vi "Read Dashboard Variables.vi"() -> ()   [LabVIEW 2018]
uses:
  <vilib>/Rock Robotics/Network Tables/NT Read Number.vi
  Framework/Robot Global Data.vi
panel:
  out "Hatch Extend Duration":dbl
  out "Hatch Extend Setpoint":dbl
  out "SlowModeSettings":i32=2
  out "MaxSpeedSlow":dbl=0.4
  out "SlowRate":dbl=1.0
  out "MaxTurnSlow":dbl=0.55
  out "MaxTurnRateSlow":dbl=20.0
  out "Cargo Stop Current":dbl
  out "Cargo Hold Duration":dbl
  out "Cheezy Drive Mode":u32=2
  out "Cargo Setpoint":dbl
  out "Elevator Duration":dbl
  out "Elevator Setpoint":dbl
  out "Pivot Right Setpoint":dbl
  out "Pivot Left Setpoint":dbl
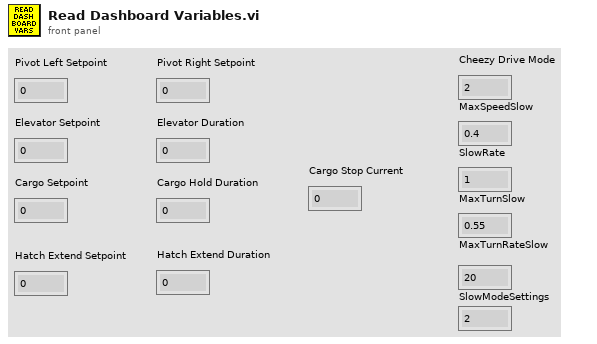
[diagram p1: front panel]
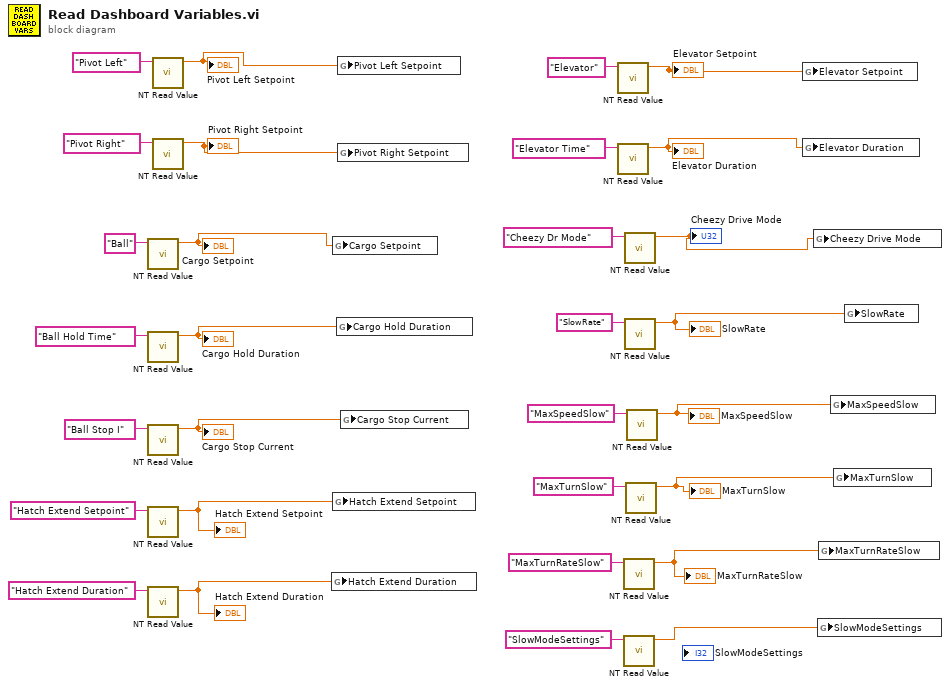
[diagram p0: block diagram]
diagram:
  n1 = call-poly <vilib>:"NT Read Value.vi"("Name"="Ball") -> ("Numeric"=w20:dbl)  [unwired: 9 in, 1 out]
  "Cargo Setpoint" <- w20
  n2 = call-poly <vilib>:"NT Read Value.vi"("Name"="Ball Hold Time") -> ("Numeric"=w18:dbl)  [unwired: 9 in, 1 out]
  "Cargo Hold Duration" <- w18
  n3 = call-poly <vilib>:"NT Read Value.vi"("Name"="Ball Stop I") -> ("Numeric"=w15:dbl)  [unwired: 9 in, 1 out]
  "Cargo Stop Current" <- w15
  n4 = call-poly <vilib>:"NT Read Value.vi"("Name"="Hatch Extend Setpoint") -> ("Numeric"=w2:dbl)  [unwired: 9 in, 1 out]
  "Hatch Extend Setpoint" <- w2
  n5 = call-poly <vilib>:"NT Read Value.vi"("Name"="Hatch Extend Duration") -> ("Numeric"=w1:dbl)  [unwired: 9 in, 1 out]
  "Hatch Extend Duration" <- w1
  n6 = call-poly <vilib>:"NT Read Value.vi"("Name"="Pivot Left") -> ("Numeric"=w24:dbl)  [unwired: 9 in, 1 out]
  "Pivot Left Setpoint" <- w24
  n7 = call-poly <vilib>:"NT Read Value.vi"("Name"="Pivot Right") -> ("Numeric"=w23:dbl)  [unwired: 9 in, 1 out]
  "Pivot Right Setpoint" <- w23
  n8 = global write "Robot Global Data.vi" "Hatch Extend Duration"(w1) -> ()
  n9 = global write "Robot Global Data.vi" "Cargo Setpoint"(w20) -> ()
  n10 = global write "Robot Global Data.vi" "Hatch Extend Setpoint"(w2) -> ()
  n11 = global write "Robot Global Data.vi" "Cargo Hold Duration"(w18) -> ()
  n12 = global write "Robot Global Data.vi" "Pivot Left Setpoint"(w24) -> ()
  n13 = global write "Robot Global Data.vi" "Pivot Right Setpoint"(w23) -> ()
  n14 = global write "Robot Global Data.vi" "Cargo Stop Current"(w15) -> ()
  n15 = call-poly <vilib>:"NT Read Value.vi"("Name"="Elevator") -> ("Numeric"=w22:dbl)  [unwired: 9 in, 1 out]
  "Elevator Setpoint" <- w22
  n16 = call-poly <vilib>:"NT Read Value.vi"("Name"="Elevator Time") -> ("Numeric"=w21:dbl)  [unwired: 9 in, 1 out]
  "Elevator Duration" <- w21
  n17 = call-poly <vilib>:"NT Read Value.vi"("Name"="MaxTurnRateSlow") -> ("Numeric"=w8:dbl)  [unwired: 9 in, 1 out]
  "MaxTurnRateSlow" <- w8
  n18 = call-poly <vilib>:"NT Read Value.vi"("Name"="SlowModeSettings") -> ("Numeric"=w6:dbl)  [unwired: 9 in, 1 out]
  n19 = call-poly <vilib>:"NT Read Value.vi"("Name"="Cheezy Dr Mode") -> ("Numeric"=w19:dbl)  [unwired: 9 in, 1 out]
  "Cheezy Drive Mode" <- w19
  n20 = call-poly <vilib>:"NT Read Value.vi"("Name"="SlowRate") -> ("Numeric"=w7:dbl)  [unwired: 9 in, 1 out]
  "SlowRate" <- w7
  n21 = call-poly <vilib>:"NT Read Value.vi"("Name"="MaxTurnSlow") -> ("Numeric"=w9:dbl)  [unwired: 9 in, 1 out]
  "MaxTurnSlow" <- w9
  n22 = call-poly <vilib>:"NT Read Value.vi"("Name"="MaxSpeedSlow") -> ("Numeric"=w10:dbl)  [unwired: 9 in, 1 out]
  "MaxSpeedSlow" <- w10
  n23 = global write "Robot Global Data.vi" "Elevator Setpoint"(w22) -> ()
  n24 = global write "Robot Global Data.vi" "Elevator Duration"(w21) -> ()
  n25 = global write "Robot Global Data.vi" "Cheezy Drive Mode"(w19) -> ()
  n26 = global write "Robot Global Data.vi" "SlowModeSettings"(w6) -> ()
  n27 = global write "Robot Global Data.vi" "MaxTurnRateSlow"(w8) -> ()
  n28 = global write "Robot Global Data.vi" "MaxSpeedSlow"(w10) -> ()
  n29 = global write "Robot Global Data.vi" "MaxTurnSlow"(w9) -> ()
  n30 = global write "Robot Global Data.vi" "SlowRate"(w7) -> ()
